vi "CLI_wrapper.vi"(8 "error in":errorcluster, 11 "exe":path=path "C:/Users/Administrator/Desktop/Azdo/emea-ni-vscd_Configurator/source/builds/ConfigurationManager/test CLI app/testCLIapp.exe") -> (0 "error out":errorcluster, 3 "result":T1)   [LabVIEW 2020]
uses:
  Shared/Controls and Global/result_type.ctl
panel:
  out "size(s)":i32
  out "mS to open":u32
  in  "return value name":string="result"
  in  "abort":bool
  in  "main VI":string="main.vi"
  in  "cmd line":string="-- /number:0"
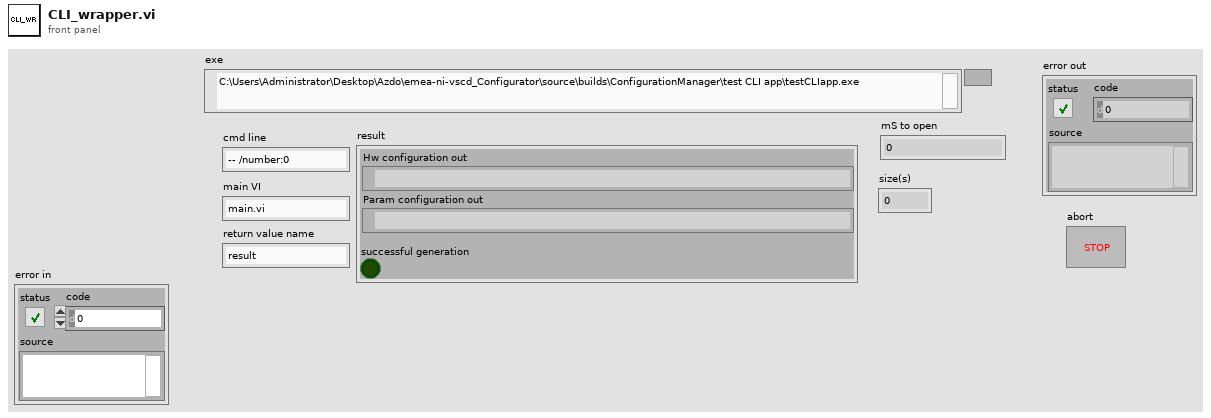
[diagram p1: front panel]
types:
  T1 = typedef "result_type.ctl" = cluster{"Hw configuration out":path, "Param configuration out":path, "successful generation":bool}
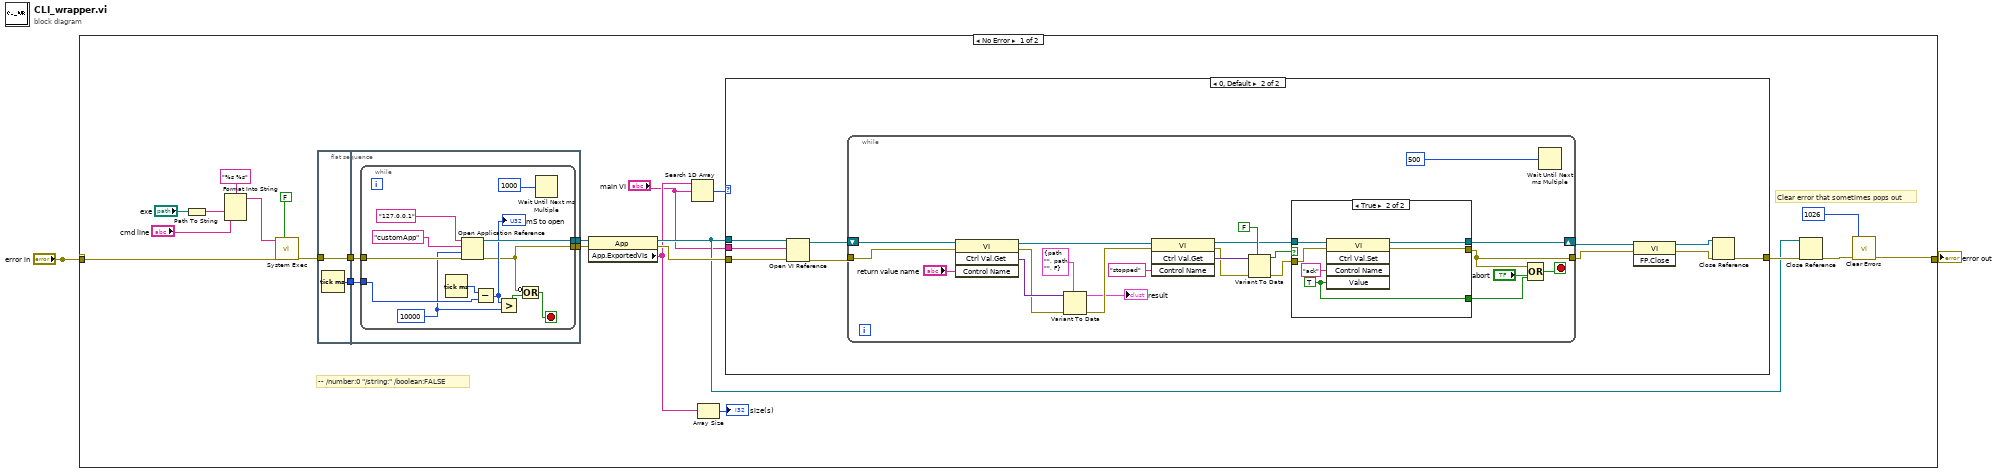
[diagram p0: block diagram]
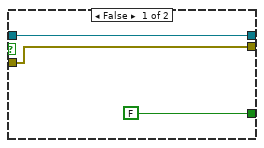
[diagram p3: hidden frame]
diagram:
  n1 = case shown="No Error" "error in" {
    selector: "error in" -> [w10 w85]
    tunnel: "error in" -> [_ _]
    tunnel: [w7 w85] -> w1
    frame No Error {
      # "Clear error that sometimes pops out"
      # "-- /number:0 \"/string:\" /boolean:FALSE"
      n2 = Path To String(path="exe") -> (string=w20:string)
      n3 = Format Into String(format string="%s %s", w20, "cmd line") -> (resulting string=w17:string)  [unwired: 2 in, 1 out]
      n4 = call <vilib>:"System Exec.vi"("wait until completion? (T)"=FALSE, "error in (no error)"=w10, "command line"=w17) -> ("error out"=w11:errorcluster)  [unwired: 5 in, 3 out]
      n5 = flat-sequence {
        tunnel: w11 -> [w26]
        tunnel: [w26] -> w24
        tunnel: [w25] -> w23
        tunnel: [w30] -> w16
        tunnel: [w29] -> w15
        tunnel: w24 -> [w28]
        tunnel: w23 -> [w27]
        frame #0 {
          n6 = Tick Count (ms)() -> (millisecond timer value=w25:u32)
        }
        frame #1 {
          n7 = while {
            tunnel: [w42] -> w30
            tunnel: [w32] -> w29
            tunnel: w28 -> [w39]
            tunnel: w27 -> [w37]
            stop <- w33 stop-if-true
            w35 = 10000 ("timeout ms (60000)")
            n8 = Tick Count (ms)() -> (millisecond timer value=w38:u32)
            n9 = Open Application Reference(8:w39, 9:w35, 10:"customApp", 11:"127.0.0.1" ("machine name (\"\":  open local reference)")) -> (0:w32:errorcluster, 3:w42:refnum<vi>)
            n10 = Subtract(x=w38, y=w37) -> (x-y=w36:u32)
            "mS to open" <- w36
            n11 = Greater?(x=w36, y=w35) -> (0:w34:bool)
            n12 = Compound Arithmetic op=OR(invert w32, w34) -> (w33:bool)
            n13 = Wait Until Next ms Multiple(millisecond multiple=u32 1000 ("millisecond timer value")) -> ()  [unwired: 1 out]
          }
        }
      }
      n14 = property class="App"(reference=w16, error in=w15) -> (reference out=w12:refnum<vi>, error out=w14:errorcluster, "App.ExportedVIs"=w5:string[])
      n15 = Search 1D Array(1D array=w5, element="main VI") -> (index of element=w3:i32)  [unwired: 1 in]
      n16 = Array Size(array=w5) -> (size(s)=→"size(s)":i32)
      n17 = case shown="0, Default" w3 {
        tunnel: w12 -> [_ w48]
        tunnel: "main VI" -> [_ w53]
        tunnel: w14 -> [w43 w52]
        tunnel: [w43 w51] -> w13
        frame -1 {
        }
        frame 0, Default {
          n18 = Open VI Reference(application reference (local)=w48, vi path=w53, error in (no error)=w52) -> (vi reference=w49:refnum<vi>, error out=w50:errorcluster)  [unwired: 3 in]
          n19 = while {
            tunnel: w50 -> [w67]
            tunnel: [w63] -> w46
            shift-right: [w61] -> w47
            shift-left: w49 -> [w68]
            stop <- w64 stop-if-true
            n20 = invoke class="VI" method="Ctrl Val.Get"(reference=w68, error in=w67, "Control Name"="return value name") -> (reference out=w66:refnum<vi>, error out=w58:errorcluster, "Get Control Value Variant"=w59:variant)  [unwired: 1 in, 1 out]
            n21 = Variant To Data(error in=w58, type=T1 {"Hw configuration out"=path "", "Param configuration out"=path "", "successful generation"=FALSE} ("result"), Variant=w59) -> (data=→"result":T1, error out=w56:errorcluster)
            n22 = invoke class="VI" method="Ctrl Val.Get"(reference=w66, error in=w56, "Control Name"="stopped") -> (reference out=w69:refnum<vi>, error out=w73:errorcluster, "Get Control Value Variant"=w74:variant)  [unwired: 1 in, 1 out]
            n23 = Variant To Data(error in=w73, type=FALSE, Variant=w74) -> (data=w71:bool, error out=w70:errorcluster)
            n24 = case shown="True" w71 {
              tunnel: w70 -> [w78 w82]
              tunnel: w69 -> [w76 w84]
              tunnel: [w78 w79] -> w63
              tunnel: [FALSE w81] -> w54
              tunnel: [w76 w80] -> w61
              frame False {
              }
              frame True {
                w81 = TRUE
                n25 = invoke class="VI" method="Ctrl Val.Set"(reference=w84, error in=w82, "Control Name"="ack", "Value"=w81) -> (reference out=w80:refnum<vi>, error out=w79:errorcluster)  [unwired: 1 in, 3 out]
              }
            }
            n26 = Compound Arithmetic op=OR(w63, "abort", w54) -> (w64:bool)
            n27 = Wait Until Next ms Multiple(millisecond multiple=500) -> ()  [unwired: 1 out]
          }
          n28 = invoke class="VI" method="FP.Close"(reference=w47, error in=w46) -> (reference out=w44:refnum<vi>, error out=w45:errorcluster)  [unwired: 1 in, 1 out]
          n29 = Close Reference(reference=w44, error in (no error)=w45) -> (error out=w51:errorcluster)
        }
      }
      n30 = Close Reference(reference=w12, error in (no error)=w13) -> (error out=w8:errorcluster)
      n31 = call <vilib>:"Clear Errors.vi"("error in (no error)"=w8, "specific error code to clear (0: all)"=1026) -> ("error out"=w7:errorcluster)  [unwired: 4 in, 1 out]
    }
    frame Error {
    }
  }
  "error out" <- w1
